vi "Exemple - SideBar.vi"() -> ()   [LabVIEW 2012]
uses:
  <vilib>/Utility/miscctls.llb/LVPointTypeDef.ctl
  Engine/Move Speed.ctl
panel:
  in  "Toolbar-Equalizer":T1={"A"=FALSE, "A 6"=FALSE, "XY Graph"=[{0.0, 1.826094800440163}, {1.0, 2.552989094122573}, {2.0, 0.018637065709899595}, {3.0, 1.5833813477750907}, {4.0, 1.3526302562966999}, {5.0, 0.6368044146170964}, {6.0, 0.7664796639047888}, {7.0, 2.4832152765458817}, {8.0, 0.8897202333846315}, {9.0, 2.340131213062037}], "Volume"=2.8804173037517833} {"Volume" scale=0.0..10.0}
  in  "Toolbar 6":T2
  in  "Toolbar 5":T3
  in  "Toolbar 4":T3
  in  "Toolbar 3":T3
  # "Move your mouse over the toolbars to reveal them."
  # "If Blocking is set to FALSE, then the Core VI will be called through VI Server \nand will not wait until the move his completed. You can see this behavior with the\ngraph in the lower left toolbar. When FALSE, the graph will refresh while moving, \notherwise, it will stop refreshing until the move is complete."
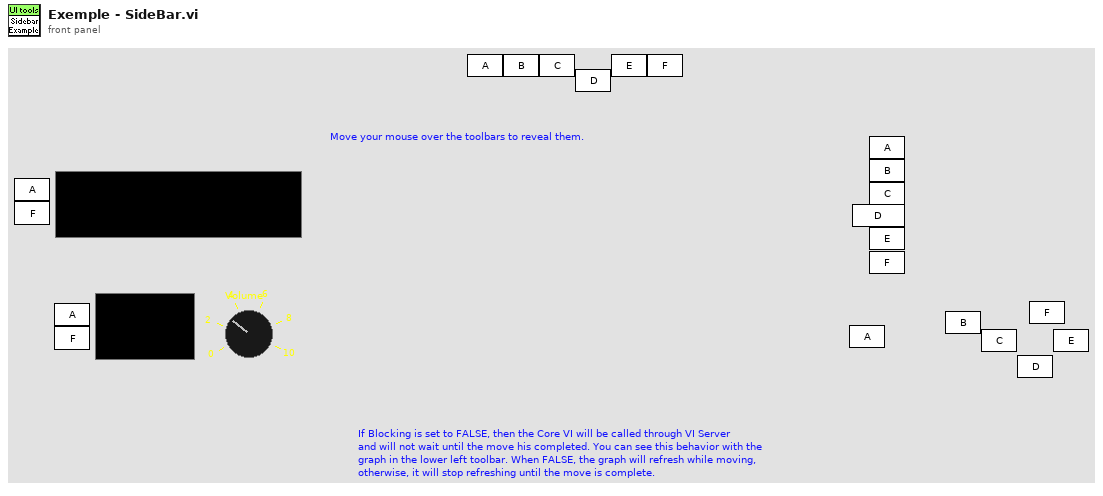
[diagram p1: front panel]
types:
  T1 = cluster{"A":bool, "A 6":bool, "XY Graph":cluster{dbl, dbl}[], "Volume":dbl}
  T2 = cluster{"A":bool, "A 6":bool, "XY Graph":cluster{dbl, dbl}[]}
  T3 = cluster{"A":bool, "A 2":bool, "A 3":bool, "A 4":bool, "A 5":bool, "A 6":bool}
  T4 = typedef "LVPointTypeDef.ctl" = cluster{"Horizontal":i16, "Vertical":i16}
  T5 = typedef "Move Speed.ctl" = enum16{"Normal", "Fast", "Slow", "Instantaneous"}
  T6 = enum32{"invalid app kind", "Development System", "Run Time System", "Student Edition", "Embedded LabVIEW", "Evaluation", "Custom"}
  T7 = typedef "LVRectTypeDef.ctl" = cluster{"Left":i16, "Top":i16, "Right":i16, "Bottom":i16}
  T8 = cluster{"left":i16, "top":i16, "right":i16, "bottom":i16}
  T9 = cluster{"left":i16, "top":i16, "right":i16, "bottom":i16}[]
  T10 = typedef "LVBoundsTypeDef.ctl" = cluster{"Width":u32, "Height":u32}
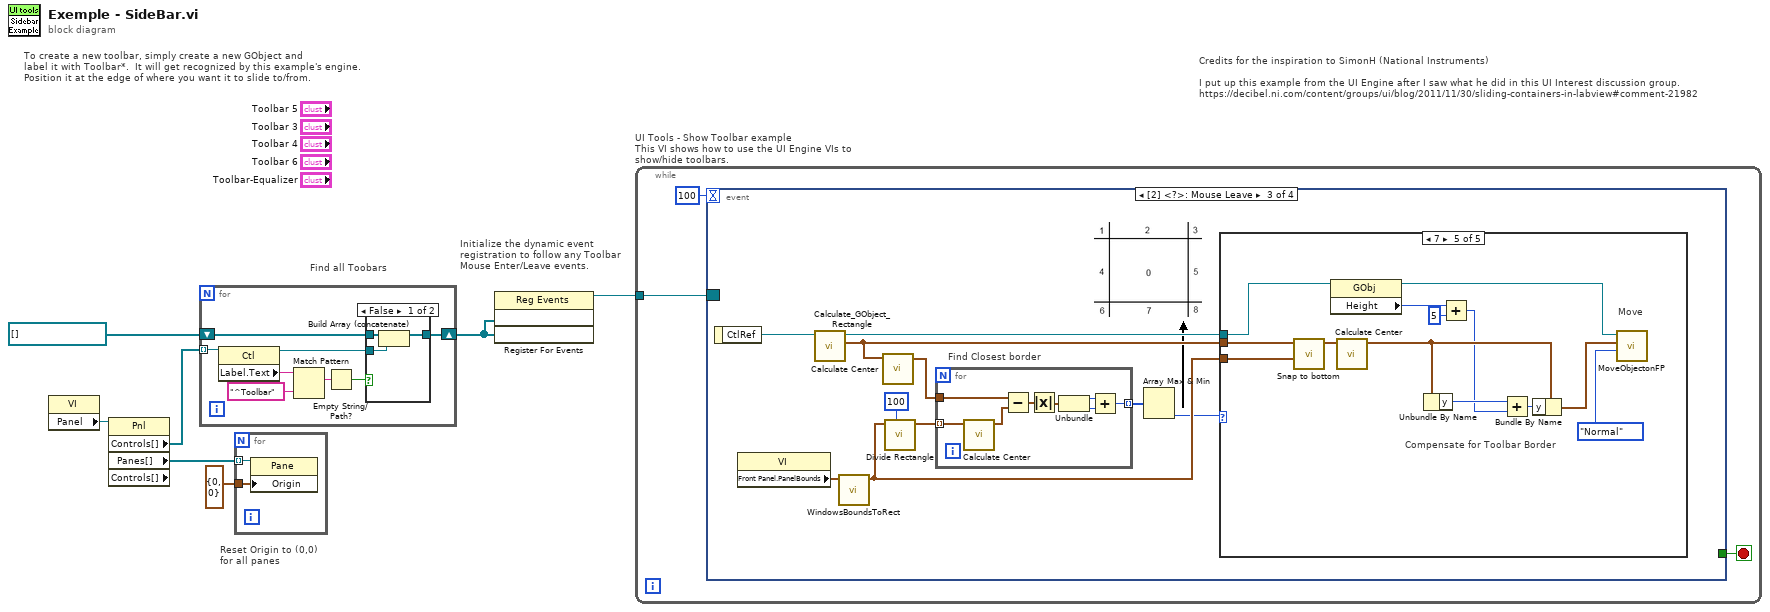
[diagram p0: block diagram]
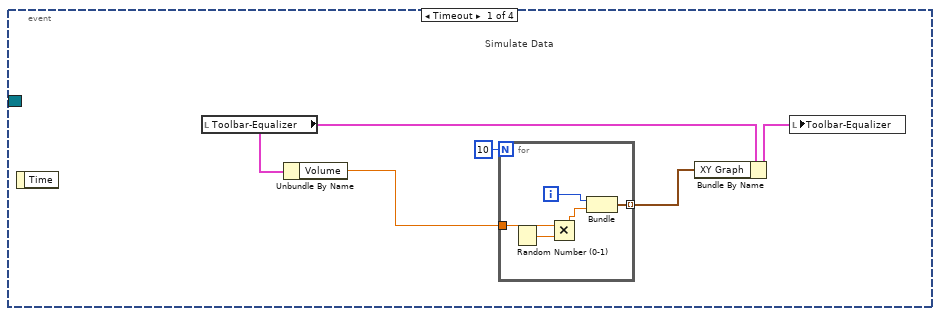
[diagram p3: hidden frame]
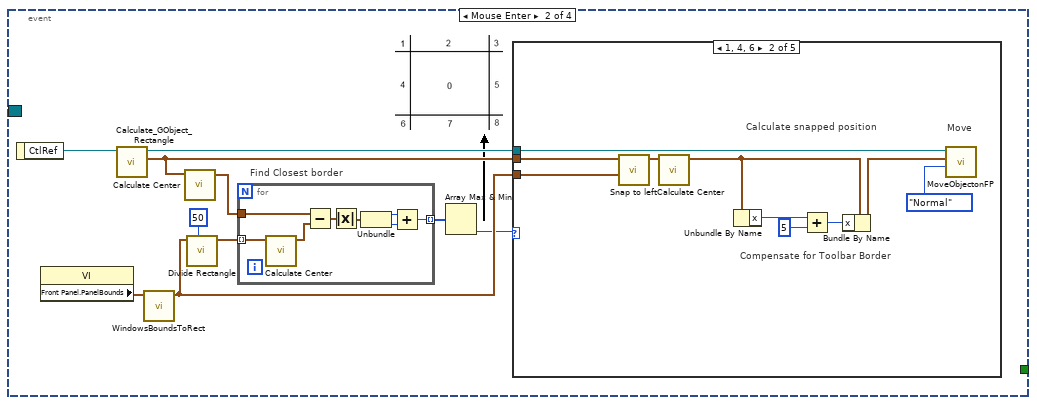
[diagram p4: hidden frame]
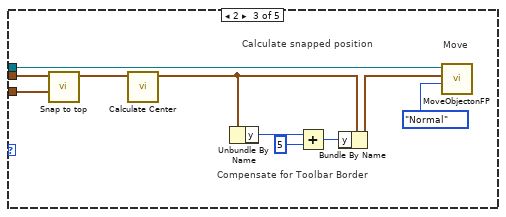
[diagram p6: hidden frame]
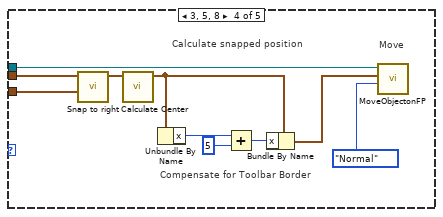
[diagram p7: hidden frame]
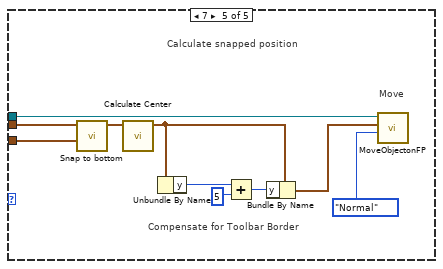
[diagram p8: hidden frame]
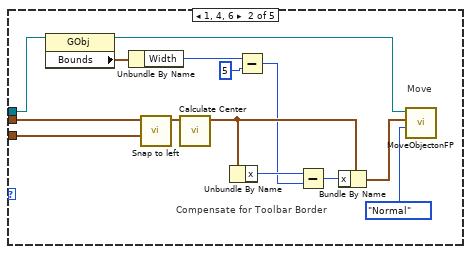
[diagram p10: hidden frame]
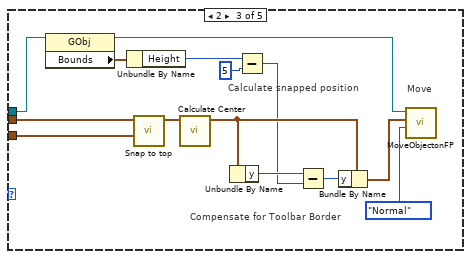
[diagram p11: hidden frame]
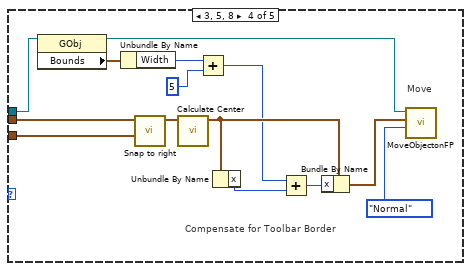
[diagram p12: hidden frame]
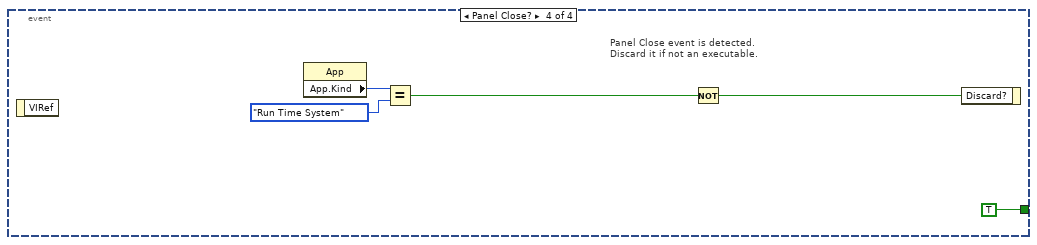
[diagram p13: hidden frame]
diagram:
  # "Credits for the inspiration to SimonH (National Instruments)\n\nI put up this example from the UI Engine after I saw what he did in this UI Interest discussion group.\nhttps://decibel.ni.com/content/groups/ui/blog/2011/11/30/sliding-containers-in-labview#comment-21982"
  # "To create a new toolbar, simply create a new GObject and \nlabel it with Toolbar*.  It will get recognized by this example's engine.\nPosition it at the edge of where you want it to slide to/from."
  # "Reset Origin to (0,0)\nfor all panes"
  # "Find all Toobars"
  # "Initialize the dynamic event\nregistration to follow any Toolbar\nMouse Enter/Leave events."
  n1 = property class="VI"() -> ("Panel"=w6:refnum<vi>)  [unwired: 2 in, 2 out]
  n2 = property class="Pnl" props=["Controls[]", "Panes[]", "Controls[]"](reference=w6) -> ("Controls[]"=w1:refnum<vi>[], "Panes[]"=w5:refnum<vi>[])  [unwired: 1 in, 3 out]
  n3 = for {
    tunnel: w1 -> [w15] mode=indexing
    shift-right: [w9] -> w2
    shift-left: refnum<vi>[] [] -> [w10]
    n4 = property class="Ctl"(reference=w15) -> (reference out=w8:refnum<vi>, "Label.Text"=w14:string)  [unwired: 1 in, 1 out]
    n5 = Match Pattern(string=w14, regular expression="^Toolbar") -> (match substring=w12:string)  [unwired: 4 out]
    n6 = Empty String/Path?(string/path=w12) -> (empty?=w11:bool)
    n7 = case shown="False" w11 {
      tunnel: [w16 w19] -> w9
      tunnel: w10 -> [w18 w19]
      tunnel: w8 -> [w17 _]
      frame False {
        n8 = Build Array (concatenate)(w18, w17) -> (w16:refnum<vi>[])
      }
      frame True {
      }
    }
  }
  n9 = for {
    tunnel: w5 -> [w21] mode=indexing
    tunnel: T4 {"Horizontal"=0, "Vertical"=0} ("Origin") -> [w20]
    n10 = property class="Pane"(reference=w21, "Origin"=w20) -> ()  [unwired: 1 in, 2 out]
  }
  n11 = register-events(w2, w2) -> (reference out=w7:refnum<event-registration>)  [unwired: 2 in, 1 out]
  n12 = while "UI Tools - Show Toolbar example\nThis VI shows how to use the UI Engine VIs to show/hide toolbars." {
    tunnel: w7 -> [w22]
    stop <- w23 stop-if-true
    n13 = event shown="[2] <?>: Mouse Leave" {
      selector: w22 -> [_ _ _ _]
      dyn-events: _ -> [_ _ _ _]
      timeout: 100 -> [_ _ _ _]
      tunnel: [_ _ _ TRUE ("Discard?")] -> w23
      event Timeout {
        # "Simulate Data"
        n14 = event-data() -> ()  [unwired: 2 out]
        n15 = local read "Toolbar-Equalizer"() -> (w28:T1)
        n16 = Unbundle By Name(w28) -> ("Volume"=w27:dbl)
        n17 = for {
          N: 10 -> [_]
          tunnel: w27 -> [w33]
          tunnel: [w30] -> w26 mode=indexing
          i -> [w32]
          n18 = Random Number (0-1)() -> (number: 0 to 1=w34:dbl)
          n19 = Multiply(x=w33, y=w34) -> (x*y=w31:dbl)
          n20 = Bundle(w32, w31) -> (w30:cluster{i32, dbl})  [unwired: 1 out]
        }
        n21 = Bundle By Name(cluster=w28, "XY Graph"=w26) -> (w29:T1)
        n22 = local write "Toolbar-Equalizer"(w29) -> ()
      }
      event Mouse Enter {
        # "Find Closest border"
        n23 = event-data() -> ("CtlRef"=w44:refnum<vi>)  [unwired: 1 out]
        n24 = property class="VI"() -> ("Front Panel.PanelBounds"=w35:T7)  [unwired: 2 in, 2 out]
        n25 = call "Calculate_GObject_Rectangle.vi"("GObject ref"=w44) -> ("Rectangle"=w41:T8, "GObject ref dup"=w36:refnum<vi>)  [unwired: 1 in, 8 out]
        n26 = call "WindowsBoundsToRect.vi"("Windows Bounds"=w35) -> ("Rectangle"=w43:T8)  [unwired: 10 out]
        n27 = call "Calculate Center.vi"("Rectangle"=w41) -> ("Center"=w39:cluster{"x":i32, "y":i32})  [unwired: 10 out]
        n28 = call "Divide Rectangle.vi"("Band (50)"=i16 50, "Rectangle"=w43) -> ("Zones Rectangles"=w40:T9)  [unwired: 1 in, 8 out]
        n29 = for {
          tunnel: w40 -> [w52] mode=indexing
          tunnel: w39 -> [w51]
          tunnel: [w45] -> w38 mode=indexing
          n30 = call "Calculate Center.vi"("Rectangle"=w52) -> ("Center"=w50:cluster{"x":i32, "y":i32})  [unwired: 10 out]
          n31 = Subtract(x=w51, y=w50) -> (x-y=w49:cluster{"x":i32, "y":i32})
          n32 = Absolute Value(x=w49) -> (abs(x)=w48:cluster{"x":i32, "y":i32})
          n33 = Unbundle(w48) -> ("x"=w47:i32, "y"=w46:i32)
          n34 = Add(x=w47, y=w46) -> (x+y=w45:i32)
        }
        n35 = Array Max & Min(array=w38) -> (min index (indices)=w37:i32)  [unwired: 3 out]
        n36 = case shown="1, 4, 6" w37 {
          tunnel: w36 -> [_ w53 w66 w81 w86]
          tunnel: w43 -> [_ w60 w64 w79 w88]
          tunnel: w41 -> [_ w59 w65 w80 w89]
          frame Default {
          }
          frame 1, 4, 6 {
            # "Compensate for Toolbar Border"
            # "Move"
            # "Calculate snapped position"
            n37 = call "Snap to left.vi"("Fixed Rect"=w60, "Rect"=w59) -> ("Snapped to left"=w61:T8)  [unwired: 1 in, 8 out]
            n38 = call "Calculate Center.vi"("Rectangle"=w61) -> ("Center"=w55:cluster{"x":i32, "y":i32})  [unwired: 10 out]
            n39 = Unbundle By Name(w55) -> ("x"=w58:i32)
            n40 = Add(x=w58, y=5) -> (x+y=w56:i32)
            n41 = Bundle By Name(cluster=w55, "x"=w56) -> (w54:cluster{"x":i32, "y":i32})
            n42 = call "MoveObjectonFP.vi"("Move Speed (Instantaneous)"=Move_Speed."Normal", "Center Position for Object"=w54, "GObject"=w53) -> ()  [unwired: 3 in, 6 out]
          }
          frame 2 {
            # "Compensate for Toolbar Border"
            # "Move"
            # "Calculate snapped position"
            n43 = call "Snap to top.vi"("Fixed Rect"=w64, "Rect"=w65) -> ("Snapped to top"=w63:T8)  [unwired: 1 in, 8 out]
            n44 = call "Calculate Center.vi"("Rectangle"=w63) -> ("Center"=w68:cluster{"x":i32, "y":i32})  [unwired: 10 out]
            n45 = Unbundle By Name(w68) -> ("y"=w71:i32)
            n46 = Add(x=w71, y=5) -> (x+y=w69:i32)
            n47 = Bundle By Name(cluster=w68, "y"=w69) -> (w67:cluster{"x":i32, "y":i32})
            n48 = call "MoveObjectonFP.vi"("Move Speed (Instantaneous)"=Move_Speed."Normal", "Center Position for Object"=w67, "GObject"=w66) -> ()  [unwired: 3 in, 6 out]
          }
          frame 3, 5, 8 {
            # "Compensate for Toolbar Border"
            # "Move"
            # "Calculate snapped position"
            n49 = call "Snap to right.vi"("Fixed Rect"=w79, "Rect"=w80) -> ("Snapped to right"=w78:T8)  [unwired: 1 in, 8 out]
            n50 = call "Calculate Center.vi"("Rectangle"=w78) -> ("Center"=w74:cluster{"x":i32, "y":i32})  [unwired: 10 out]
            n51 = Unbundle By Name(w74) -> ("x"=w77:i32)
            n52 = Add(x=w77, y=5) -> (x+y=w75:i32)
            n53 = Bundle By Name(cluster=w74, "x"=w75) -> (w73:cluster{"x":i32, "y":i32})
            n54 = call "MoveObjectonFP.vi"("Move Speed (Instantaneous)"=Move_Speed."Normal", "Center Position for Object"=w73, "GObject"=w81) -> ()  [unwired: 3 in, 6 out]
          }
          frame 7 {
            # "Compensate for Toolbar Border"
            # "Move"
            # "Calculate snapped position"
            n55 = call "Snap to bottom.vi"("Fixed Rect"=w88, "Rect"=w89) -> ("Snapped to bottom"=w87:T8)  [unwired: 1 in, 8 out]
            n56 = call "Calculate Center.vi"("Rectangle"=w87) -> ("Center"=w84:cluster{"x":i32, "y":i32})  [unwired: 10 out]
            n57 = Unbundle By Name(w84) -> ("y"=w91:i32)
            n58 = Add(x=w91, y=5) -> (x+y=w90:i32)
            n59 = Bundle By Name(cluster=w84, "y"=w90) -> (w83:cluster{"x":i32, "y":i32})
            n60 = call "MoveObjectonFP.vi"("Move Speed (Instantaneous)"=Move_Speed."Normal", "Center Position for Object"=w83, "GObject"=w86) -> ()  [unwired: 3 in, 6 out]
          }
        }
      }
      event Mouse Leave {
        # "Find Closest border"
        n61 = event-data() -> ("CtlRef"=w94:refnum<vi>)  [unwired: 1 out]
        n62 = property class="VI"() -> ("Front Panel.PanelBounds"=w93:T7)  [unwired: 2 in, 2 out]
        n63 = call "Calculate_GObject_Rectangle.vi"("GObject ref"=w94) -> ("Rectangle"=w99:T8, "GObject ref dup"=w102:refnum<vi>)  [unwired: 1 in, 8 out]
        n64 = call "WindowsBoundsToRect.vi"("Windows Bounds"=w93) -> ("Rectangle"=w101:T8)  [unwired: 10 out]
        n65 = call "Calculate Center.vi"("Rectangle"=w99) -> ("Center"=w97:cluster{"x":i32, "y":i32})  [unwired: 10 out]
        n66 = call "Divide Rectangle.vi"("Band (50)"=i16 100, "Rectangle"=w101) -> ("Zones Rectangles"=w98:T9)  [unwired: 1 in, 8 out]
        n67 = for {
          tunnel: w98 -> [w110] mode=indexing
          tunnel: w97 -> [w109]
          tunnel: [w103] -> w96 mode=indexing
          n68 = call "Calculate Center.vi"("Rectangle"=w110) -> ("Center"=w108:cluster{"x":i32, "y":i32})  [unwired: 10 out]
          n69 = Subtract(x=w109, y=w108) -> (x-y=w107:cluster{"x":i32, "y":i32})
          n70 = Absolute Value(x=w107) -> (abs(x)=w106:cluster{"x":i32, "y":i32})
          n71 = Unbundle(w106) -> ("x"=w105:i32, "y"=w104:i32)
          n72 = Add(x=w105, y=w104) -> (x+y=w103:i32)
        }
        n73 = Array Max & Min(array=w96) -> (min index (indices)=w95:i32)  [unwired: 3 out]
        n74 = case shown="7" w95 {
          tunnel: w102 -> [_ w115 w132 w145 w157]
          tunnel: w101 -> [_ w122 w126 w150 w161]
          tunnel: w99 -> [_ w121 w127 w151 w162]
          frame Default {
          }
          frame 1, 4, 6 {
            # "Compensate for Toolbar Border"
            # "Move"
            n75 = property class="GObj"(reference=w115) -> (reference out=w114:refnum<vi>, "Bounds"=w116:T10)  [unwired: 1 in, 1 out]
            n76 = Unbundle By Name(w116) -> ("Width"=w113:u32)
            n77 = call "Snap to left.vi"("Fixed Rect"=w122, "Rect"=w121) -> ("Snapped to left"=w123:T8)  [unwired: 1 in, 8 out]
            n78 = call "Calculate Center.vi"("Rectangle"=w123) -> ("Center"=w118:cluster{"x":i32, "y":i32})  [unwired: 10 out]
            n79 = Unbundle By Name(w118) -> ("x"=w120:i32)
            n80 = Subtract(x=w113, y=u32 5) -> (x-y=w111:u32)
            n81 = Subtract(x=w120, y=w111) -> (x-y=w119:u32)
            n82 = Bundle By Name(cluster=w118, "x"=w119) -> (w117:cluster{"x":i32, "y":i32})
            n83 = call "MoveObjectonFP.vi"("Move Speed (Instantaneous)"=Move_Speed."Normal", "Center Position for Object"=w117, "GObject"=w114) -> ()  [unwired: 3 in, 6 out]
          }
          frame 2 {
            # "Compensate for Toolbar Border"
            # "Move"
            # "Calculate snapped position"
            n84 = property class="GObj"(reference=w132) -> (reference out=w131:refnum<vi>, "Bounds"=w133:T10)  [unwired: 1 in, 1 out]
            n85 = Unbundle By Name(w133) -> ("Height"=w130:u32)
            n86 = call "Snap to top.vi"("Fixed Rect"=w126, "Rect"=w127) -> ("Snapped to top"=w125:T8)  [unwired: 1 in, 8 out]
            n87 = call "Calculate Center.vi"("Rectangle"=w125) -> ("Center"=w135:cluster{"x":i32, "y":i32})  [unwired: 10 out]
            n88 = Unbundle By Name(w135) -> ("y"=w137:i32)
            n89 = Subtract(x=w130, y=u32 5) -> (x-y=w128:u32)
            n90 = Subtract(x=w137, y=w128) -> (x-y=w136:u32)
            n91 = Bundle By Name(cluster=w135, "y"=w136) -> (w134:cluster{"x":i32, "y":i32})
            n92 = call "MoveObjectonFP.vi"("Move Speed (Instantaneous)"=Move_Speed."Normal", "Center Position for Object"=w134, "GObject"=w131) -> ()  [unwired: 3 in, 6 out]
          }
          frame 3, 5, 8 {
            # "Compensate for Toolbar Border"
            # "Move"
            n93 = property class="GObj"(reference=w145) -> (reference out=w144:refnum<vi>, "Bounds"=w146:T10)  [unwired: 1 in, 1 out]
            n94 = Unbundle By Name(w146) -> ("Width"=w141:u32)
            n95 = call "Snap to right.vi"("Fixed Rect"=w150, "Rect"=w151) -> ("Snapped to right"=w149:T8)  [unwired: 1 in, 8 out]
            n96 = call "Calculate Center.vi"("Rectangle"=w149) -> ("Center"=w148:cluster{"x":i32, "y":i32})  [unwired: 10 out]
            n97 = Add(x=w141, y=5) -> (x+y=w139:u32)
            n98 = Unbundle By Name(w148) -> ("x"=w143:i32)
            n99 = Add(x=w139, y=w143) -> (x+y=w142:u32)
            n100 = Bundle By Name(cluster=w148, "x"=w142) -> (w147:cluster{"x":i32, "y":i32})
            n101 = call "MoveObjectonFP.vi"("Move Speed (Instantaneous)"=Move_Speed."Normal", "Center Position for Object"=w147, "GObject"=w144) -> ()  [unwired: 3 in, 6 out]
          }
          frame 7 {
            # "Compensate for Toolbar Border"
            # "Move"
            n102 = call "Snap to bottom.vi"("Fixed Rect"=w161, "Rect"=w162) -> ("Snapped to bottom"=w160:T8)  [unwired: 1 in, 8 out]
            n103 = property class="GObj"(reference=w157) -> (reference out=w156:refnum<vi>, "Height"=w159:u32)  [unwired: 1 in, 1 out]
            n104 = call "Calculate Center.vi"("Rectangle"=w160) -> ("Center"=w164:cluster{"x":i32, "y":i32})  [unwired: 10 out]
            n105 = Unbundle By Name(w164) -> ("y"=w154:i32)
            n106 = Add(x=w159, y=u32 5) -> (x+y=w153:u32)
            n107 = Add(x=w154, y=w153) -> (x+y=w155:u32)
            n108 = Bundle By Name(cluster=w164, "y"=w155) -> (w163:cluster{"x":i32, "y":i32})
            n109 = call "MoveObjectonFP.vi"("Move Speed (Instantaneous)"=Move_Speed."Normal", "Center Position for Object"=w163, "GObject"=w156) -> ()  [unwired: 3 in, 6 out]
          }
        }
      }
      event Panel Close? {
        # "Panel Close event is detected.\nDiscard it if not an executable."
        n110 = event-data() -> ()  [unwired: 2 out]
        n111 = property class="App"() -> ("App.Kind"=w169:T6)  [unwired: 2 in, 2 out]
        n112 = Equal?(x=w169, y=T6."Run Time System" ("Application:Kind")) -> (x = y?=w168:bool)
        n113 = Not(x=w168) -> (.not. x?=w166:bool)
        n114 = event-data("Discard?"=w166) -> ()  [unwired: 1 in, 1 out]
      }
    }
  }
